vi "Config file functional global for GUIs.vi"(7 "GUI elements":T1, 8 "error in":errorcluster, 9 "text to write":string, 10 "file path":path, 11 "Mode":T2=enum."Rewrite file") -> (0 "error out":errorcluster, 1 "text read":string, 2 "file path":path, 3 "NaN/Path/Refnum?":bool)   [LabVIEW 2010]
doc: "This .vi handles interactions with the config file (which stores the front panel values) for the various GUI elements (MAIN.vi, SLM Utility, AO tree, etc.)"
uses:
  HHMI - Config file functional global mode enum.ctl
  User interface config file selector enum.ctl
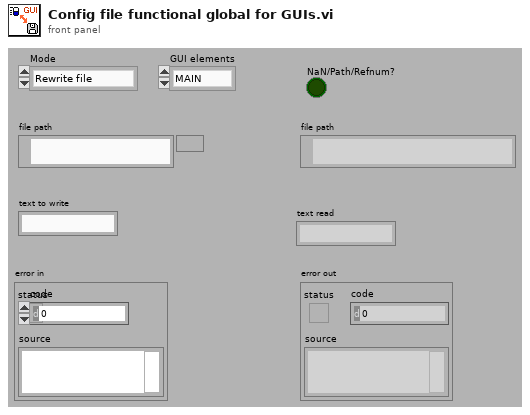
[diagram p1: front panel]
types:
  T1 = typedef "User interface config file selector enum.ctl" = enum16{"MAIN"}
  T2 = typedef "HHMI - Config file functional global mode enum.ctl" = enum16{"Set Filepath", "Read file", "Rewrite file"}
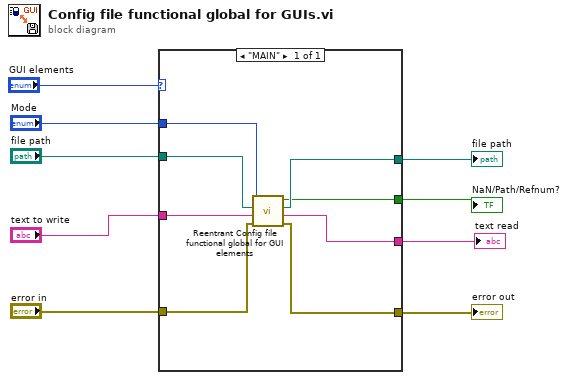
[diagram p0: block diagram]
diagram:
  n1 = case shown="\"MAIN\"" "GUI elements" {
    tunnel: "Mode" -> [w17]
    tunnel: "error in" -> [w16]
    tunnel: [w15] -> w7
    tunnel: "text to write" -> [w14]
    tunnel: [w13] -> w5
    tunnel: [w12] -> w4
    tunnel: "file path" -> [w11]
    tunnel: [w10] -> w2
    frame "MAIN" {
      n2 = call "Reentrant Config file functional global for GUI elements.vi"("error in"=w16, "text to write"=w14, "file path"=w11, "Mode"=w17) -> ("error out"=w15:errorcluster, "text read"=w13:string, "file path"=w12:path, "Not a Refnum?"=w10:bool)  [unwired: 2 in, 2 out]
    }
  }
  "file path" <- w4
  "error out" <- w7
  "NaN/Path/Refnum?" <- w2
  "text read" <- w5
